vi "ALTS-2015 Simulation DataSocket URL.vi"(3 "Update rate (100 ms)":u32=100, 4 "Item Name":string) -> (0 "URL":string)   [LabVIEW 2013]
panel:
  # "Create an OPC URL from Several Inputs"
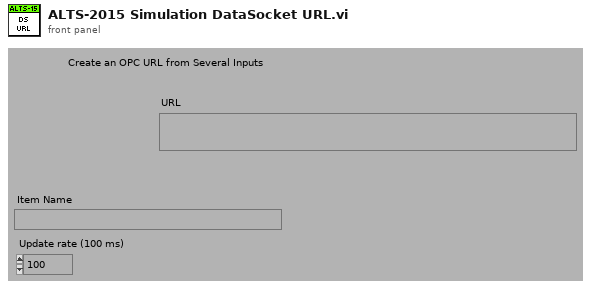
[diagram p1: front panel]
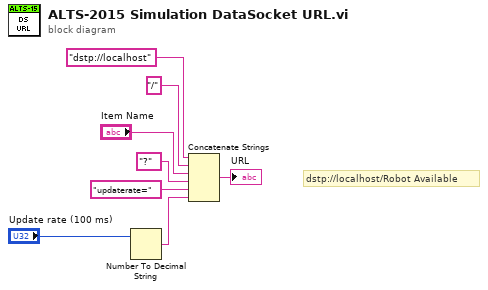
[diagram p0: block diagram]
diagram:
  # "dstp://localhost/Robot Available"
  n1 = Number To Decimal String(number="Update rate (100 ms)") -> (decimal integer string=w5:string)  [unwired: 1 in]
  n2 = Concatenate Strings("dstp://localhost", "/", "Item Name", "?", "updaterate=", w5) -> (→"URL":string)
